vi "AUTOFOCUS_init.vi"(1 "variant":variant, 5 "Dimension size":i32, 7 "MCL Handle":i32, 9 "channel":bool, 11 "error in":errorcluster) -> (2 "Init":bool, 3 "Y initialized array":dbl[](array[numeric]), 4 "X initialized array":dbl[](array[numeric]), 6 "Z0":dbl, 8 "Autotune":bool, 10 "Setpoint":dbl, 12 "Switch":bool, 13 "QPDcount OUT":u32, 14 "PID cluster":T1, 15 "error out":errorcluster)   [LabVIEW 2015]
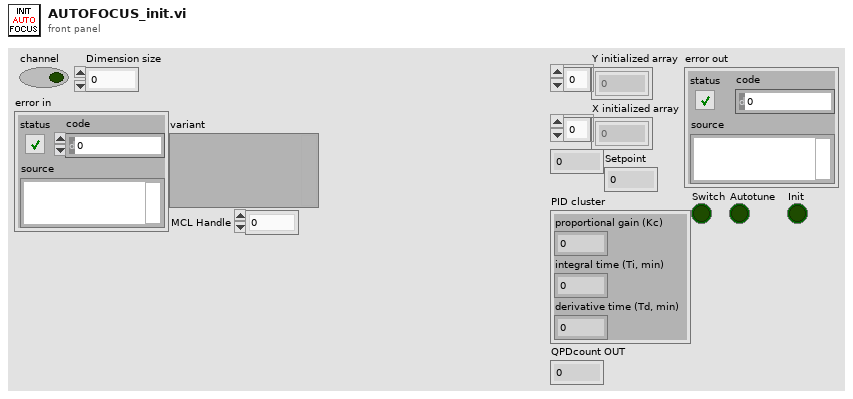
[diagram p1: front panel]
types:
  T1 = cluster{"proportional gain (Kc)":dbl, "integral time (Ti, min)":dbl, "derivative time (Td, min)":dbl}
  T2 = cluster{"Init":bool, "Switch":bool, "Autotune?":bool, "PID gains":cluster{"proportional gain (Kc)":dbl, "integral time (Ti, min)":dbl, "derivative time (Td, min)":dbl}}
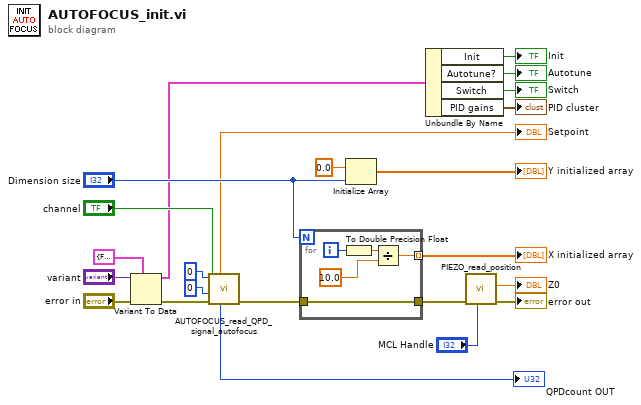
[diagram p0: block diagram]
diagram:
  n1 = Variant To Data(error in="error in", type=T2 {"Init"=FALSE, "Switch"=FALSE, "Autotune?"=FALSE, "PID gains"={"proportional gain (Kc)"=0.0, "integral time (Ti, min)"=0.0, "derivative time (Td, min)"=0.0}} ("output cluster"), Variant="variant") -> (data=w12:T2, error out=w8:errorcluster)
  n2 = call "AUTOFOCUS_read_QPD_signal_autofocus.vi"("error in"=w8, "i IR lost"=0, "channel"="channel", "QPDcount"=u32 0) -> ("error out"=w23:errorcluster, "QPDcount OUT"=→"QPDcount OUT":u32, "QPD"=→"Setpoint":dbl)  [unwired: 1 in, 2 out]
  n3 = for {
    N: "Dimension size" -> [_]
    tunnel: [w26] -> w17 mode=indexing
    tunnel: w23 -> [w25]
    tunnel: [w25] -> w22
    i -> [w28]
    n4 = To Double Precision Float(number=w28) -> (double precision float=w24:dbl)
    n5 = Divide(x=w24, y=10.0) -> (x/y=w26:dbl)
  }
  "X initialized array" <- w17
  n6 = Initialize Array(0.0 ("element"), "Dimension size") -> (→"Y initialized array":dbl[])
  n7 = Unbundle By Name(w12) -> ("Init"=→"Init":bool, "Autotune?"=→"Autotune":bool, "Switch"=→"Switch":bool, "PID gains"=→"PID cluster":T1)
  n8 = call "PIEZO_read_position.vi"("MCL Handle"="MCL Handle", "error MCL in"=w22) -> ("error MCL out"=→"error out":errorcluster, "Z piezo"=→"Z0":dbl)  [unwired: 6 in, 2 out]
